vi "SerialComm.vi"(8 "error in (no error)":errorcluster, 10 "Write Command":string="0R0!", 11 "VISA Refnum in":refnum<visa-resource-name>) -> (0 "error out":errorcluster, 2 "Read Buffer":string, 3 "VISA Refnum out":refnum<visa-resource-name>)   [LabVIEW 2015]
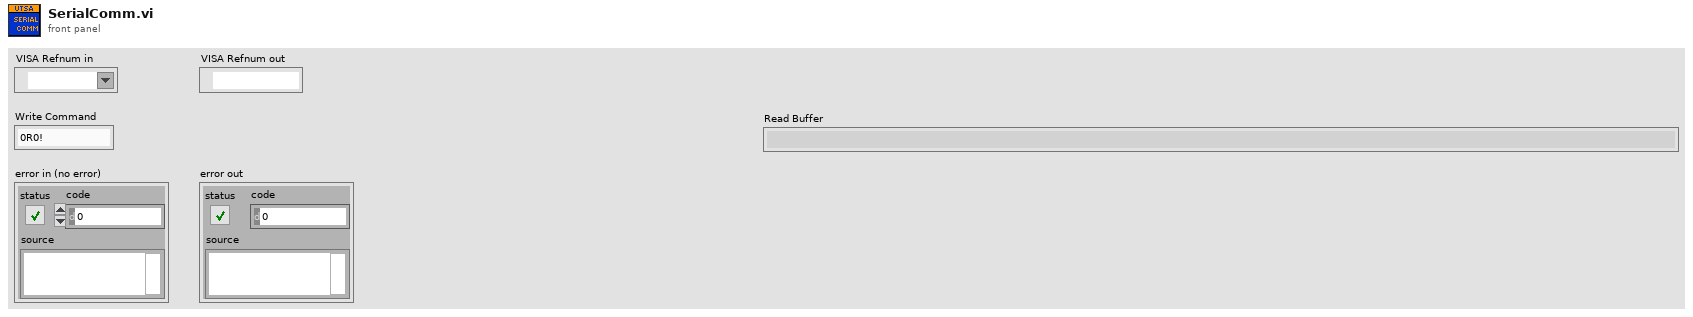
[diagram p1: front panel]
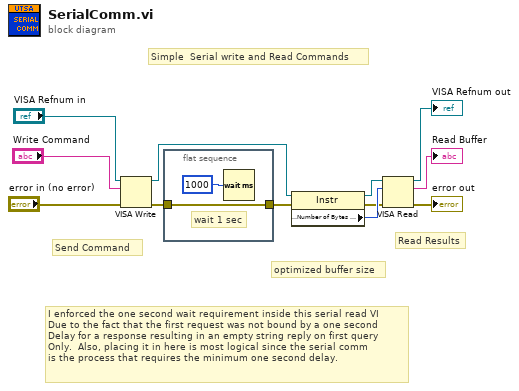
[diagram p0: block diagram]
diagram:
  # "optimized buffer size"
  # "I enforced the one second wait requirement inside this serial read VI \nDue to the fact that the first request was not bound by a one second\nDelay for a response resulting in an empty string reply on first query \nOnly.  Also, placing it in here is most logical since the serial comm\nis the process that requires the minimum one second delay."
  # "Read Results"
  # "Send Command"
  # "Simple  Serial write and Read Commands"
  n1 = VISA Write(VISA resource name="VISA Refnum in", write buffer="Write Command", error in (no error)="error in (no error)") -> (VISA resource name out=w6:refnum<visa-resource-name>, error out=w2:errorcluster)  [unwired: 1 out]
  n2 = flat-sequence {
    tunnel: w2 -> [w13]
    tunnel: [w13] -> w1
    frame #0 {
      # "wait 1 sec"
      n3 = Wait (ms)(milliseconds to wait=u32 1000 ("millisecond multiple")) -> ()  [unwired: 1 out]
    }
  }
  n4 = property class="Instr"(reference=w6, error in=w1) -> (reference out=w8:refnum<visa-resource-name>, error out=w9:errorcluster, "Serial Settings:Number of Bytes at Serial Port"=w10:u32)
  n5 = VISA Read(VISA resource name=w8, byte count=w10, error in (no error)=w9) -> (VISA resource name out=→"VISA Refnum out":refnum<visa-resource-name>, read buffer=→"Read Buffer":string, error out=→"error out":errorcluster)  [unwired: 1 out]
